vi "_Find SheetData.vi"(8 "error in":errorcluster, 10 "Worksheet":refnum<k24>) -> (0 "error out":errorcluster, 2 "SheetData":refnum<k24>)   [LabVIEW 2021, in "Open Xml.lvlib"]
uses:
  Open Xml.lvlib
  D:/git/Open-Xml-LabVIEW/DocumentFormat.OpenXml.dll
  DocumentFormat.OpenXml.dll
  D:/git/Open-Xml-LabVIEW/DocumentFormat.OpenXml.Framework.dll
  DocumentFormat.OpenXml.Framework.dll
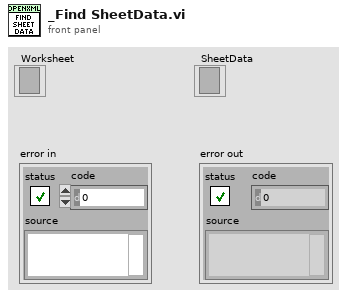
[diagram p1: front panel]
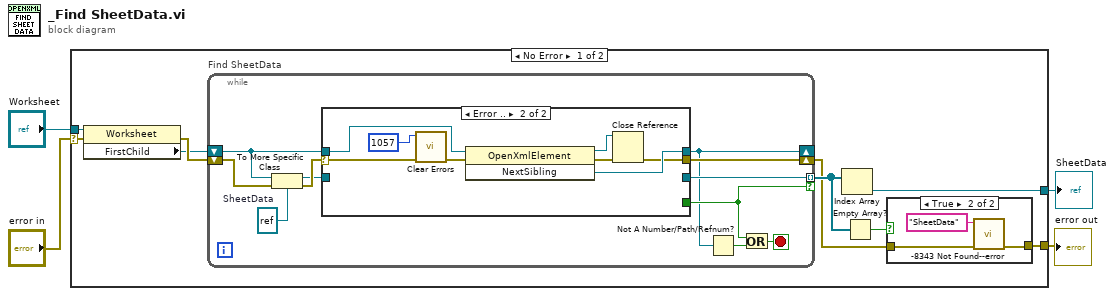
[diagram p0: block diagram]
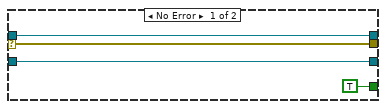
[diagram p2: hidden frame]
diagram:
  n1 = case shown="No Error" "error in" {
    selector: "error in" -> [w10 w41]
    tunnel: "Worksheet" -> [w11 _]
    tunnel: [w8 _] -> w2
    tunnel: [w5 w41] -> w1
    frame No Error {
      n2 = property class="Worksheet"(reference=w11, error in=w10) -> (error out=w13:errorcluster, "FirstChild"=w12:refnum<k24>)  [unwired: 1 out]
      n3 = while "Find SheetData" {
        shift-right: [w23] -> w6
        shift-left: w13 -> [w24]
        shift-right: [w14] -> _
        shift-left: w12 -> [w18]
        tunnel: [w16] -> w9 mode=indexing if=w15
        stop <- w19 stop-if-true
        w20 = refnum<k24> refnum  # SheetData
        n4 = To More Specific Class(target class=w20, reference=w18, error in=w24) -> (specific class reference=w17:refnum<k24>, error out=w21:errorcluster)
        n5 = case shown="Error .." w21 {
          selector: w21 -> [w28 w33]
          tunnel: [w28 w30] -> w23
          tunnel: [w25 w32] -> w14
          tunnel: [TRUE _] -> w15
          tunnel: w18 -> [w25 w31]
          tunnel: w17 -> [w26 _]
          tunnel: [w26 _] -> w16
          frame No Error {
          }
          frame Error {
            n6 = call <vilib>:"Clear Errors.vi"("error in (no error)"=w33, "specific error code to clear (0: all)"=1057) -> ("error out"=w35:errorcluster)  [unwired: 4 in, 1 out]
            n7 = invoke class="OpenXmlElement" method="NextSibling"(reference=w31, error in=w35) -> (reference out=w29:refnum<k24>, error out=w36:errorcluster, "NextSibling"=w32:refnum<k24>)  [unwired: 1 in]
            n8 = Close Reference(reference=w29, error in (no error)=w36) -> (error out=w30:errorcluster)
          }
        }
        n9 = Not A Number/Path/Refnum?(number/path/refnum=w14) -> (NaN/Path/Refnum?=w22:bool)
        n10 = Or(x=w15, y=w22) -> (x .or. y?=w19:bool)
      }
      n11 = Index Array(array=w9) -> (element=w8:refnum<k24>)  [unwired: 1 in]
      n12 = Empty Array?(array=w9) -> (empty?=w7:bool)
      n13 = case shown="True" w7 {
        tunnel: w6 -> [w37 w40]
        tunnel: [w37 w39] -> w5
        frame False {
        }
        frame True {
          n14 = call "-8343 Not Found--error.vi"("error in (no error)"=w40, "Item"="SheetData") -> ("error out"=w39:errorcluster)  [unwired: 9 in]
        }
      }
    }
    frame Error {
    }
  }
  "error out" <- w1
  "SheetData" <- w2
